vi "GPIB Send Message.vi"(2 "timeout ms":u32=4294967295 format="%.0x", 3 "address string":string, 4 "write buffer":string, 7 "source":string, 8 "write mode (set END:0)":i32(ring) items=["send EOI with last character of string", "append CR to string and send EOI with CR", "append LF to string and send EOI with LF", "append CR LF to string and send EOI with LF", "append CR to string but do not send EOI", "append LF to string but do not send EOI", "append CR LF to string but do not send EOI", "do not send EOI"], 9 "error in":T1) -> (1 "byte count":i32, 5 "status":bool[](array[boolean]), 6 "error out":T1)   [LabVIEW 2013]
doc: "Sends a string to a message based instrument."
panel:
  in  "[empty array]":bool[](array[boolean])
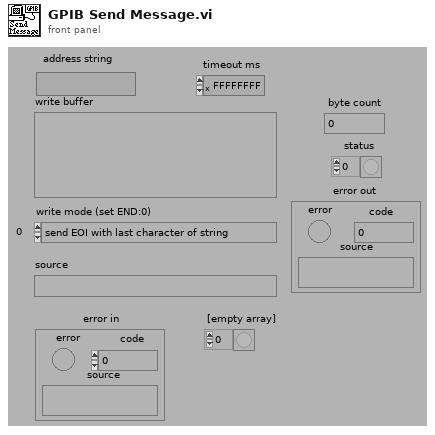
[diagram p1: front panel]
types:
  T1 = cluster{"error":bool, "code":i32, "source":string}
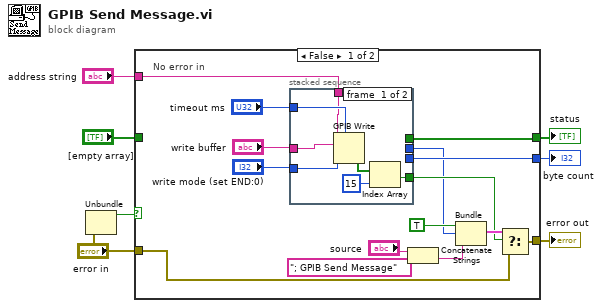
[diagram p0: block diagram]
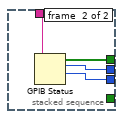
[diagram p2: hidden frame]
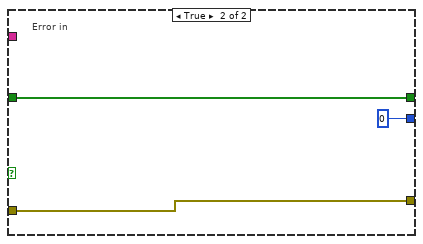
[diagram p3: hidden frame]
diagram:
  n1 = Unbundle("error in") -> ("error"=w3:bool)  [unwired: 2 out]
  n2 = case shown="False" w3 {
    tunnel: "[empty array]" -> [_ w34]
    tunnel: [w15 w34] -> w4
    tunnel: [w21 w35] -> w5
    tunnel: "error in" -> [w12 w35]
    tunnel: [w16 0] -> w7
    tunnel: "address string" -> [w8 _]
    frame False {
      # "No error in"
      n3 = stacked-sequence {
        tunnel: [_ w32] -> w15
        tunnel: [_ w33] -> w16
        tunnel: [w26 _] -> w17
        tunnel: "write mode (set END:0)" -> [w24 _]
        tunnel: "write buffer" -> [w27 _]
        tunnel: [_ w31] -> w14
        tunnel: "timeout ms" -> [w25 _]
        tunnel: w8 -> [w23 w30]
        frame #0 {
          n4 = GPIB Write(0:w23, 1:w27, 2:w24, 4:w25) -> (5:w28:bool[])  [unwired: 1 in, 1 out]
          n5 = Index Array(array=w28, index=15) -> (element=w26:bool)
        }
        frame #1 {
          n6 = GPIB Status(0:w30) -> (2:w32:bool[], 3:w31:i16, 4:w33:i32)  [unwired: 1 in, 1 out]
        }
      }
      n7 = Concatenate Strings("source", "; GPIB Send Message") -> (w13:string)
      n8 = Bundle(TRUE, "GPIB error"=w14, w13) -> (w22:cluster{bool, "GPIB error":i16, string})  [unwired: 1 in]
      n9 = Select(t=w22, s=w17, f=w12) -> (s? t:f=w21:T1)
    }
    frame True {
      # "Error in"
    }
  }
  "status" <- w4
  "error out" <- w5
  "byte count" <- w7
